vi "Msg.vi"(7 "Actor in":refnum<class "Actor.lvclass">, 11 "Actor Last Ack Msg Strategy in":refnum<class "Actor Last Ack Msg Strategy.lvclass">) -> (0 "error out":errorcluster, 5 "Actor out":refnum<class "Actor.lvclass">)   [LabVIEW 2021, in "Actor Last Ack.lvlib" / "Actor Last Ack Msg Strategy.lvclass"]
uses:
  Actor Last Ack Msg Strategy.lvclass
  LVCAM/Actor/Actor.lvclass
  Actor Last Ack/Actor Last Ack.lvclass
  Actor Last Ack Msg Strategy.lvclass/Actor Last Ack Msg Strategy.ctl
  000b8c16-d1b9-4729-a321-6082ffefced5.vi
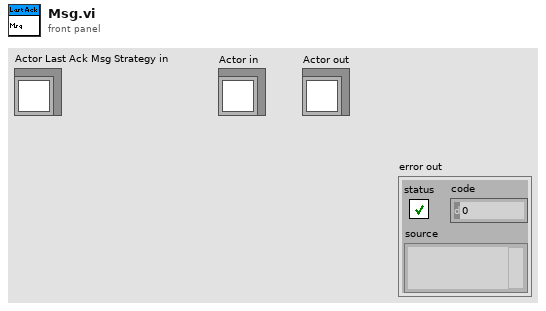
[diagram p1: front panel]
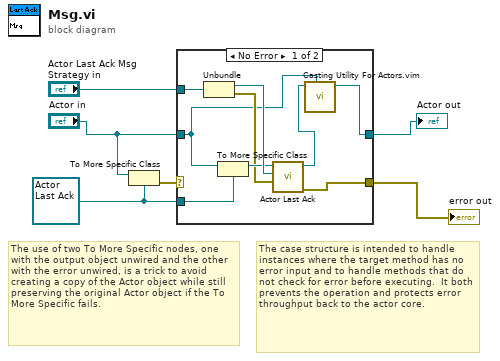
[diagram p0: block diagram]
diagram:
  w1 = refnum<class "Actor Last Ack.lvclass"> refnum ("Last Ack.lvlib:Last Ack.lvclass")
  # "The use of two To More Specific nodes, one with the output object unwired and the other with the error unwired, is a trick to avoid creating a copy of the Actor object while still preserving the original Actor object if the To More Specific fails."
  # "The case structure is intended to handle instances where the target method has no error input and to handle methods that do not check for error before executing.  It both prevents the operation and protects error throughput back to the actor core."
  n1 = To More Specific Class(target class=w1, reference="Actor in") -> (error out=w6:errorcluster)  [unwired: 1 in, 1 out]
  n2 = case shown="No Error" w6 {
    selector: w6 -> [_ w17]
    tunnel: [w13 w17] -> w4
    tunnel: [w7 w16] -> w2
    tunnel: "Actor in" -> [w8 w16]
    tunnel: "Actor Last Ack Msg Strategy in" -> [w15 _]
    tunnel: w1 -> [w11 _]
    frame No Error {
      n3 = Unbundle(w15) -> (w14:refnum<class "Actor.lvclass">, w10:errorcluster)
      n4 = To More Specific Class(target class=w11, reference=w8) -> (specific class reference=w12:refnum<class "Actor Last Ack.lvclass">)  [unwired: 1 in, 1 out]
      n5 = call-dynamic "Actor Last Ack.vi"("Nest Error"=w10, "Nest Actor"=w14, "Actor Last Ack in"=w12) -> ("error out"=w13:errorcluster, "Actor Last Ack out"=w9:refnum<class "Actor Last Ack.lvclass">)  [unwired: 7 in]
      n6 = call "Casting Utility For Actors.vim"("type"=w8, "Actor in"=w9) -> ("Actor out"=w7:refnum<class "Actor.lvclass">)  [unwired: 8 in, 1 out]
    }
    frame Error {
      # "If type check fails, pass the original object out again."
    }
  }
  "error out" <- w4
  "Actor out" <- w2
